vi "2014 Target Detection.vi"(10 "Image Ctl Refnum":refnum<vi>, 11 "Image in":T1) -> (0 "Mask":T1(plugin-control), 2 "Image Out":T1(plugin-control), 3 "Target Info":T6(array[cluster]))   [LabVIEW 2013]
uses:
  <vilib>/Rock Robotics/WPI/Camera/WPI_CameraSettings Read MJPG.ctl
  <vilib>/Rock Robotics/WPI/Camera/WPI_CameraImageSize.ctl
  TargetType.ctl
  <vilib>/vision/Image Controls.llb/IMAQ Image.ctl
panel:
  in  "Instructions:":string="Images:\nUse the tab immediately below to choose the image source. Update the camera settings or the image directory so that you have images or video to test with.\n\nCalibration:\nYou can update Color Component ranges directly, or by clicking and drawing a line on the colored strip in the Image control. The Std Dev multipliers and where the strip is drawn determine the calibration values.\n\nUse Debugging tab to view the result of the color range threshold .\n\nArea Size LImit is used to ignore objects too small or far away to care about.\n\nThe Details tab contains score details for each target and subObject.\n\nCamera Type is used to select lens angles for distance calculation.\n\nVertical strips with no adjacent horizontal strip are identified as \"not hot\" and marked in blue.\nThe numeric scores indicate represent aspect ratio and rectangularity.\n\nWhen both strips are near enough, the pair is identified as \"hot\" and marked in green. Scores\nindicate the left, right, ratio of widths, and vertical positioning.\n\nAny score that falls below cutoff is drawn in red and bounding box is drawn in red."
  in  "Std Devs":cluster{"Hue":dbl, "Sat":dbl, "Val":dbl}={"Hue"=4.0, "Sat"=6.0, "Val"=4.0}
  in  "Area Size Limit %":dbl=0.06 format="%#_13g"
  in  "Camera Type":enum16{"206", "1011", "1013"}(ring)=enum."1013"
  out "loop time ms":u32
  in  "Score Cutoff":dbl(slide)=54.248366013071895 scale=0.0..100.0
  in  "Color Components":T2={"Hue"={70.81028747558594, 157.43295288085938}, "Sat"={0.0, 255.0}, "Val"={237.4729766845703, 255.0}} {"Val" scale=0.0..255.0; "Sat" scale=0.0..255.0; "Hue" scale=0.0..255.0 scale format="%#_3g"}
  out "Error":bool
  in  "Image Source":enum32{"Files", "Camera"}(tab)
  in  "List of image files":i32(listbox)
  in  "Image Directory":path=path "2014 Pseudo-Target/2014 Pseudo-Target Active"
  in  "Camera Settings":T3={"fps"=15, "compression"=5, "Image Size"=enum."320x240"}
  in  "Camera IP":string="10.00.00.11"
  in  "Tabbed Info":enum32{"Debugging", "Details"}(tab)
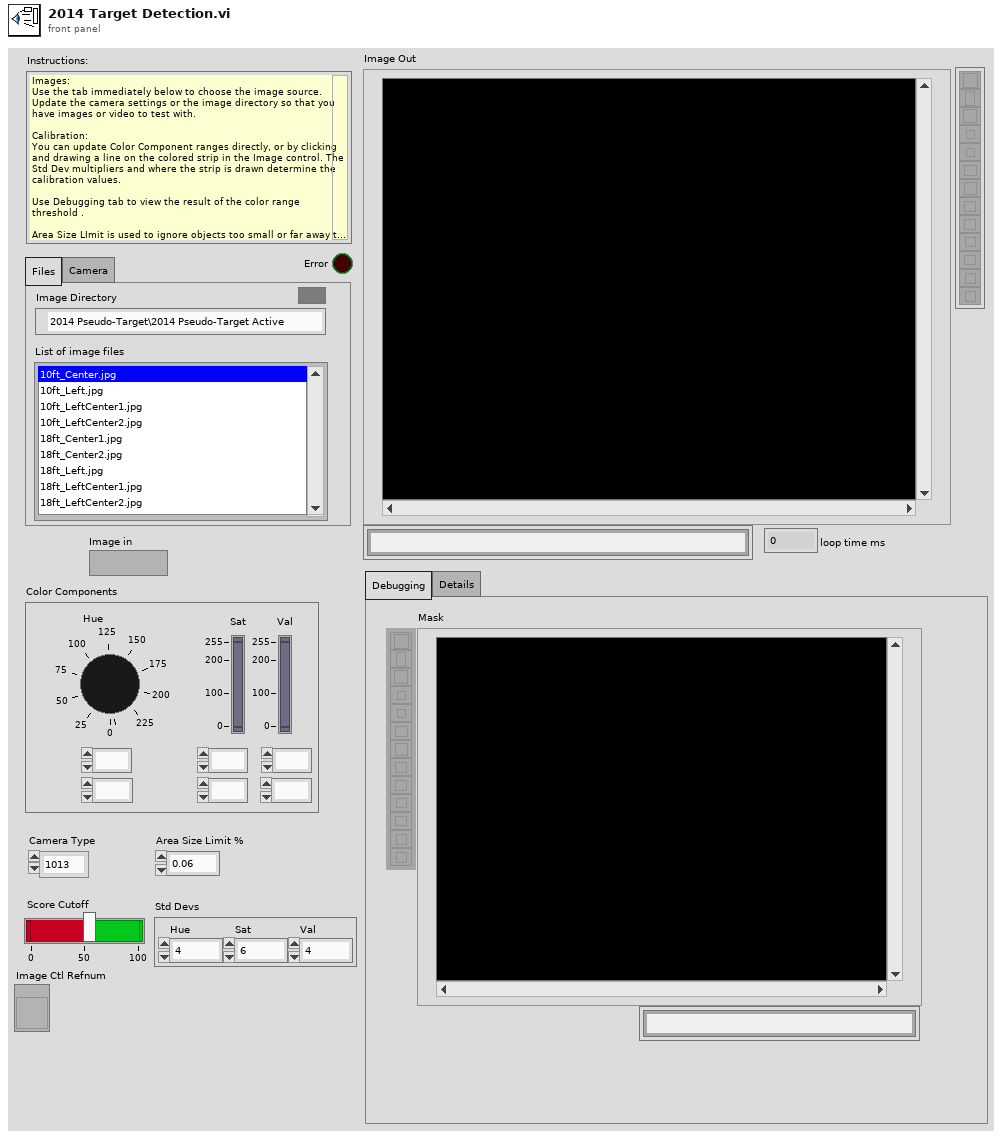
[diagram p1: front panel]
types:
  T1 = typedef "IMAQ Image.ctl" = refnum<image>
  T2 = cluster{"Hue":cluster{dbl, dbl}, "Sat":cluster{dbl, dbl}, "Val":cluster{dbl, dbl}}
  T3 = typedef "WPI_CameraSettings Read MJPG.ctl" = cluster{"fps":i32, "compression":i32, "Image Size":T4}
  T4 = typedef "WPI_CameraImageSize.ctl" = enum16{"640x480", "320x240", "160x120"}
  T5 = typedef "TargetType.ctl" = enum16{"Not Hot", "Hot"}
  T6 = cluster{"Scores":cluster{"Total":dbl, "Left":dbl, "Right":dbl, "Ratio":dbl, "Vertical":dbl, "index":i32, "State":T5}, "Verticals":cluster{"Horizontal?":bool, "Aspect Score":dbl, "Rect Score":dbl, cluster{"Left":dbl, "Top":dbl, "Right":dbl, "Bottom":dbl}, "Equiv H":dbl, "Equiv V":dbl}, "Horizontals":cluster{"Horizontal?":bool, "Aspect Score":dbl, "Rect Score":dbl, cluster{"Left":dbl, "Top":dbl, "Right":dbl, "Bottom":dbl}, "Equiv H":dbl, "Equiv V":dbl}, "Distance ft":dbl, "Center":cluster{"X":dbl, "Y":dbl}}[]
  T7 = cluster{"Horizontal":bool, "Aspect Score":dbl, "Rect Score":dbl, cluster{"Left":dbl, "Top":dbl, "Right":dbl, "Bottom":dbl}, "Equiv H":dbl, "Equiv V":dbl}[]
  T8 = cluster{cluster{dbl, dbl}, cluster{dbl, dbl}, cluster{dbl, dbl}}
  T9 = cluster{"Scores":cluster{"Total":dbl, "Left":dbl, "Right":dbl, "Ratio":dbl, "Vertical":dbl, "index":i32, "State":T5}, "Verticals":cluster{"Horizontal?":bool, "Aspect Score":dbl, "Rect Score":dbl, cluster{"Left":dbl, "Top":dbl, "Right":dbl, "Bottom":dbl}, "Equiv H":dbl, "Equiv V":dbl}, "Horizontals":cluster{"Horizontal?":bool, "Aspect Score":dbl, "Rect Score":dbl, cluster{"Left":dbl, "Top":dbl, "Right":dbl, "Bottom":dbl}, "Equiv H":dbl, "Equiv V":dbl}, "Validated":bool}[]
  T10 = cluster{"Scores":cluster{"Total":dbl, "Left":dbl, "Right":dbl, "Ratio":dbl, "Vertical":dbl, "index":i32, "State":T5}, "Verticals":cluster{"Horizontal?":bool, "Aspect Score":dbl, "Rect Score":dbl, cluster{"Left":dbl, "Top":dbl, "Right":dbl, "Bottom":dbl}, "Equiv H":dbl, "Equiv V":dbl}, "Horizontals":cluster{"Horizontal?":bool, "Aspect Score":dbl, "Rect Score":dbl, cluster{"Left":dbl, "Top":dbl, "Right":dbl, "Bottom":dbl}, "Equiv H":dbl, "Equiv V":dbl}, "Distance (ft)":dbl, "Target Center (-1 to 1)":cluster{"X":dbl, "Y":dbl}}[]
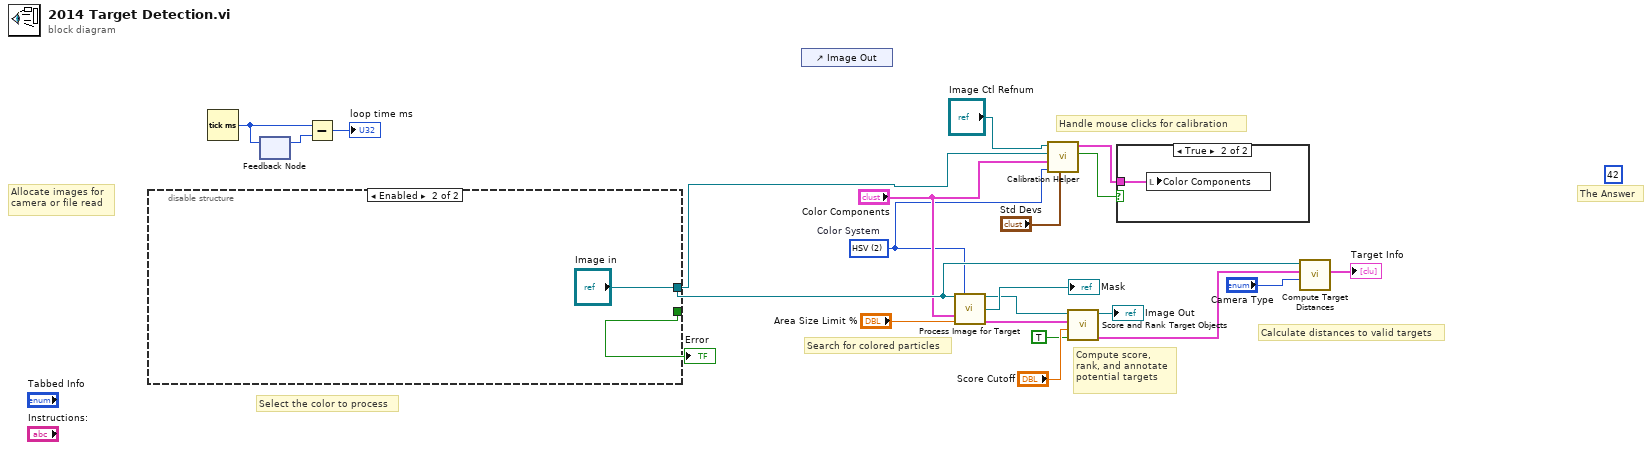
[diagram p0: block diagram]
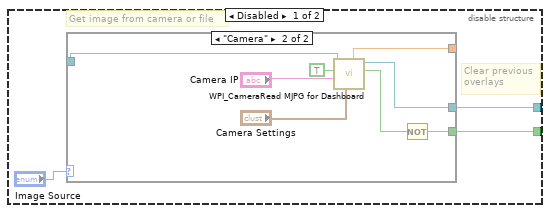
[diagram p2: hidden frame]
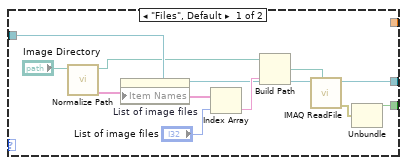
[diagram p3: hidden frame]
diagram:
  (unwired) 42
  w4 = u16 2 items=["RGB", "HSL", "HSV", "HSI"]  # Color System
  # "The Answer"
  # "Calculate distances to valid targets"
  # "Search for colored particles"
  # "Handle mouse clicks for calibration"
  # "Compute score,\nrank, and annotate\npotential targets"
  # "Select the color to process"
  # "Allocate images for\ncamera or file read"
  n1 = disable-structure shown="Enabled" {
    disable-tunnel: [w25 "Image in"] -> w6
    disable-tunnel: [w22 _] -> w21
    frame Disabled {
      # "Clear previous\noverlays"
      # "Get image from camera or file"
      n2 = case shown="\"Camera\"" "Image Source" {
        tunnel: [w32 w42] -> w25
        tunnel: [w31 w43] -> w23
        tunnel: [w29 w37] -> w22
        tunnel: [_ w36] -> _
        frame "Files", Default {
          n3 = call "Normalize Path.vi"("Image Directory"="Image Directory") -> ("Filenames"=w27:string[], "Path"=w26:path)  [unwired: 9 in]
          n4 = property on="List of image files" class="LstBox (strict)"("Item Names"=w27) -> ()  [unwired: 2 in, 2 out]
          n5 = Index Array(array=w27, index="List of image files") -> (element=w34:string)
          n6 = Build Path(base path=w26, name or relative path=w34) -> (appended path=w33:path)
          n7 = call "IMAQ ReadFile"("File Path"=w33, "Image"=w31) -> ("error out"=w30:errorcluster, "Image Out"=w32:T1)  [unwired: 5 in, 3 out]
          n8 = Unbundle(w30) -> ("status"=w29:bool)  [unwired: 2 out]
        }
        frame "Camera" {
          n9 = call <vilib>:"WPI_CameraRead MJPG for Dashboard.vi"("Camera Settings"="Camera Settings", "Camera IP"="Camera IP", "Enable"=TRUE, "Refnum in"=w43) -> ("Active"=w39:bool, "Refnum out"=w42:T1, "Bandwidth (Mbps)"=w36:dbl)  [unwired: 4 in, 1 out]
          n10 = Not(x=w39) -> (.not. x?=w37:bool)
        }
      }
    }
    frame Enabled {
    }
  }
  "Error" <- w21
  n11 = Tick Count (ms)() -> (millisecond timer value=w20:u32)
  n12 = feedback #1() -> (w19:u32)  [unwired: 1 in]
  n13 = feedback-in #1(w20) -> ()
  n14 = Subtract(x=w20, y=w19) -> (x-y=→"loop time ms":u32)
  n15 = control-ref of="Image Out"() -> ()  [unwired: 1 out]
  n16 = call "Process Image for Target.vi"("Src Image"=w6, "Color Mode"=w4, "Color Components"="Color Components", "Area Cutoff %"="Area Size Limit %") -> ("Src Image Out"=w15:T1, "Threshold"=→"Mask":T1, "Particles"=w12:T7)  [unwired: 9 in]
  n17 = call "Calibration Helper.vi"("Std Devs"="Std Devs", "Color Mode"=w4, "Color Components"="Color Components", "Image"=w6, "Image Ctl Refnum"="Image Ctl Refnum") -> ("Changed"=w3:bool, "output color"=w2:T8)  [unwired: 5 in]
  n18 = call "Score and Rank Target Objects.vi"("Annotate"=TRUE, "Score Limit"="Score Cutoff", "Particles"=w12, "Image in"=w15) -> ("Target Info"=w11:T9, "Annotated Image"=→"Image Out":T1)  [unwired: 6 in]
  n19 = case shown="True" w3 {
    tunnel: w2 -> [_ w45]
    frame False {
    }
    frame True {
      n20 = local write "Color Components"(w45) -> ()
    }
  }
  n21 = call "Compute Target Distances.vi"("Camera Type"="Camera Type", "Target Info"=w11, "Image in"=w6) -> ("Target Info"=→"Target Info":T10)  [unwired: 6 in, 2 out]
